vi "FTW-Inbox-Core-LoadMessageRouterPrototype.vi"(11 "error in":errorcluster) -> (4 "Message Router Prototype":refnum<vi>, 15 "error out":errorcluster)   [LabVIEW 2015]
panel:
  # "Inputs"
  # "Outputs"
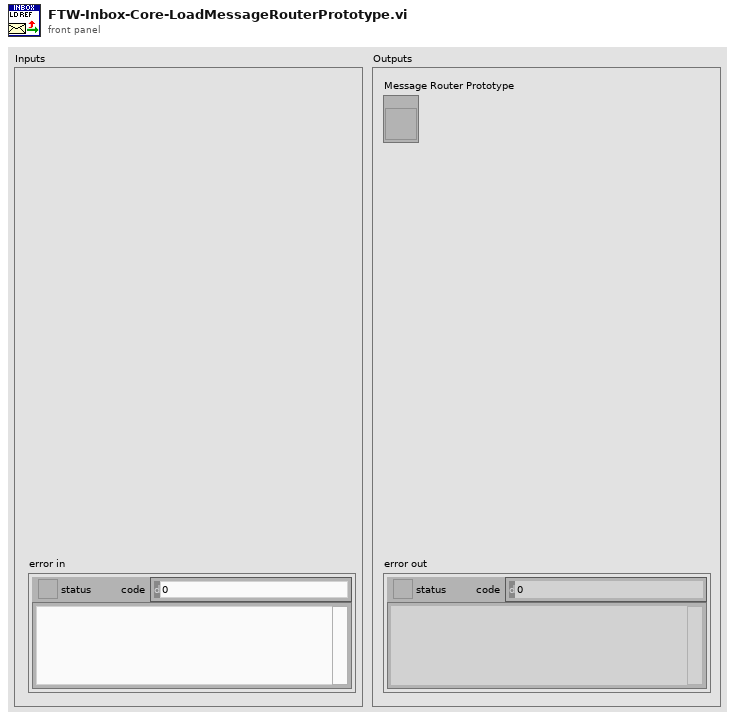
[diagram p1: front panel]
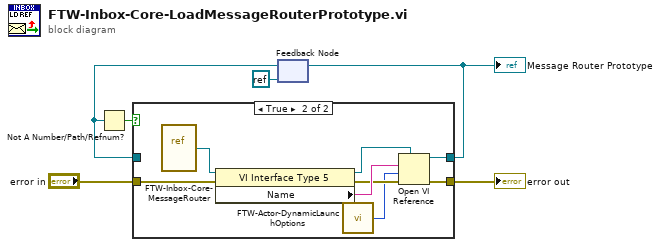
[diagram p0: block diagram]
diagram:
  n1 = feedback #1(refnum<k0> refnum) -> (w5:refnum<vi>)
  n2 = Not A Number/Path/Refnum?(number/path/refnum=w5) -> (NaN/Path/Refnum?=w4:bool)
  n3 = case shown="True" w4 {
    tunnel: [w7 w11] -> w6
    tunnel: [w8 w10] -> w2
    tunnel: "error in" -> [w8 w9]
    tunnel: w5 -> [w7 _]
    frame False {
    }
    frame True {
      n4 = vi-ref "FTW-Inbox-Core-MessageRouter.vi"() -> (w12:refnum<vi>)
      n5 = property class="VI Interface Type 5"(reference=w12, error in=w9) -> (reference out=w15:refnum<vi>, error out=w14:errorcluster, "Name"=w16:string)
      n6 = call "FTW-Actor-DynamicLaunchOptions.vi"() -> ("Open VI Ref Options"=w13:i32)  [unwired: 1 in]
      n7 = Open VI Reference(type specifier VI Refnum (for type only)=w15, vi path=w16, options=w13, error in (no error)=w14) -> (vi reference=w11:refnum<vi>, error out=w10:errorcluster)  [unwired: 2 in]
    }
  }
  "error out" <- w2
  "Message Router Prototype" <- w6
  n8 = feedback-in #1(w6) -> ()
